vi "Set pump parameters.vi"(4 "Pump write delay (ms)":dbl=300.0, 5 "Volume (uL)":dbl, 6 "Rate (uL/h)":dbl, 7 "Units":dbl=3.0, 8 "Pump #":dbl=1.0, 9 "Pump Parameters In":T1, 10 "VISA resource name":refnum<visa-resource-name>="COM4") -> (3 "Pump Parameters Out":T1)   [LabVIEW 2014]
panel:
  out "F-format string 4":string
  out "F-format string 2":string
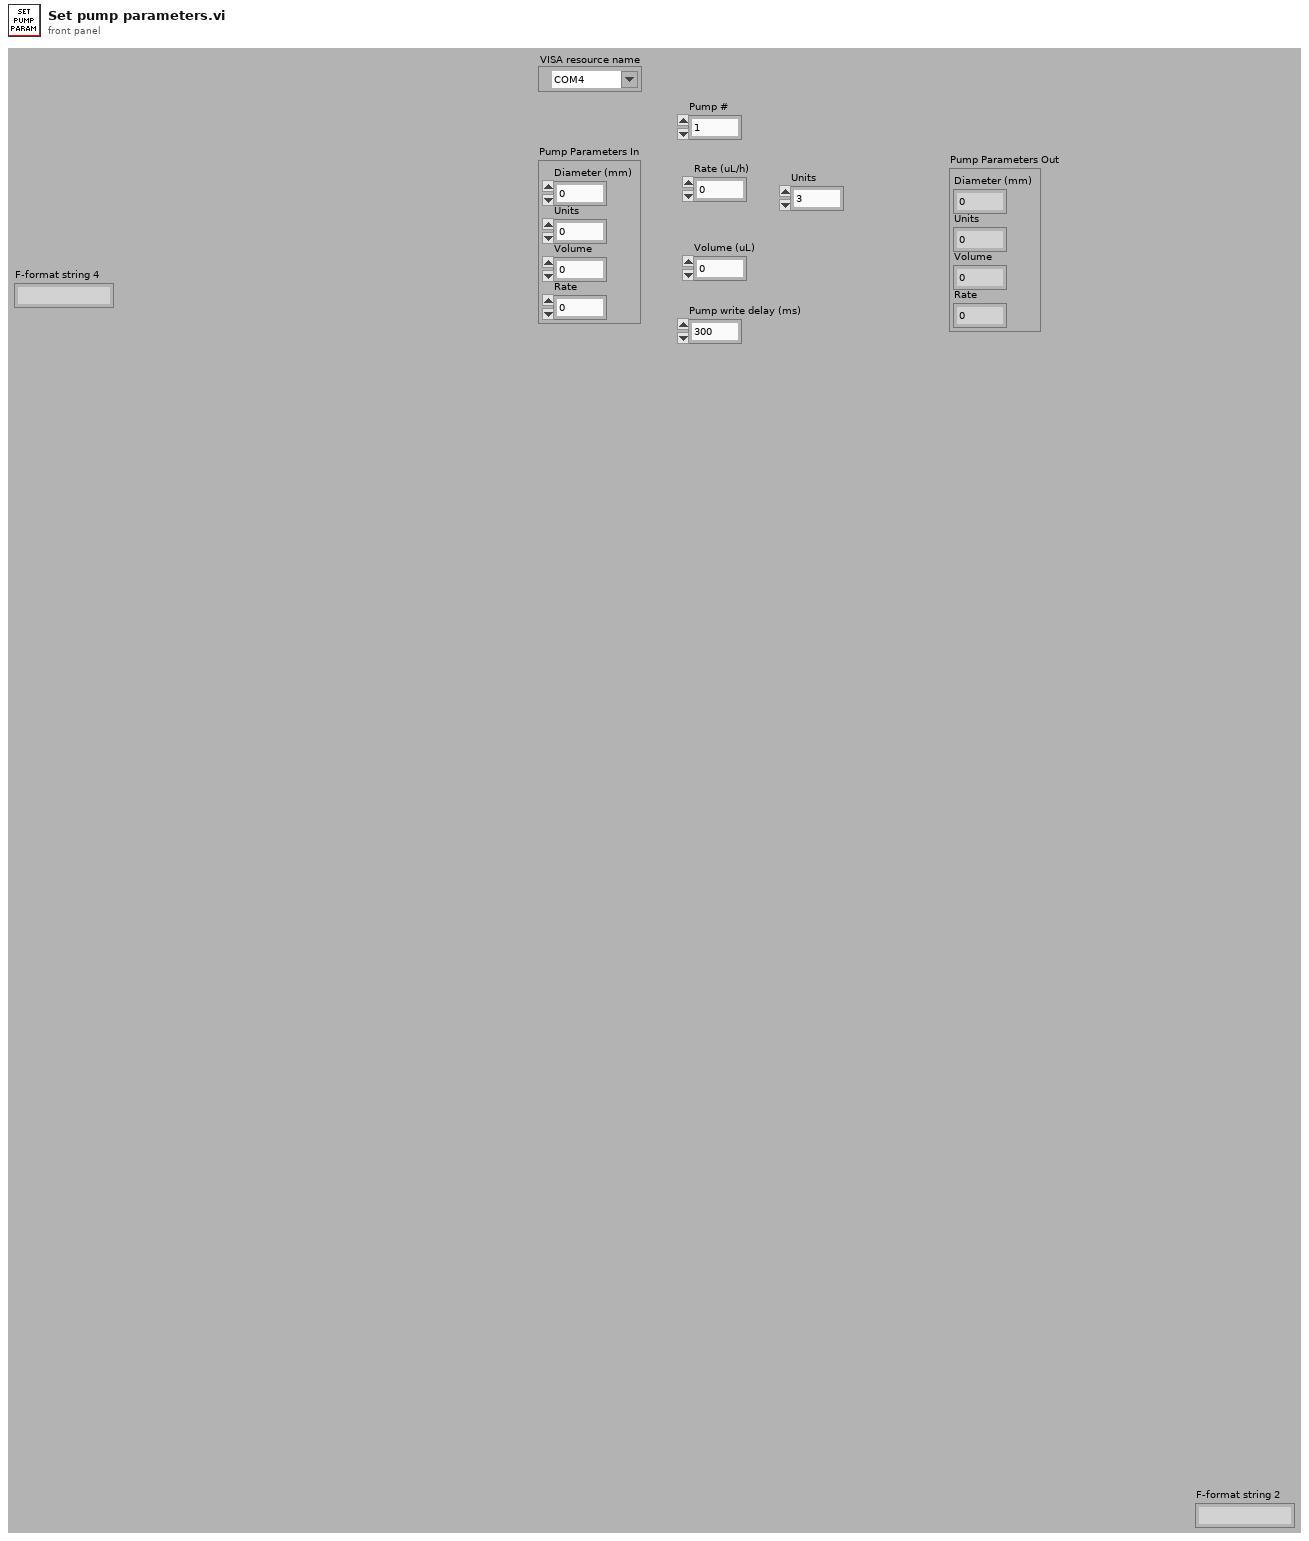
[diagram p1: front panel]
types:
  T1 = cluster{"Diameter (mm)":dbl, "Units":dbl, "Volume":dbl, "Rate":dbl}
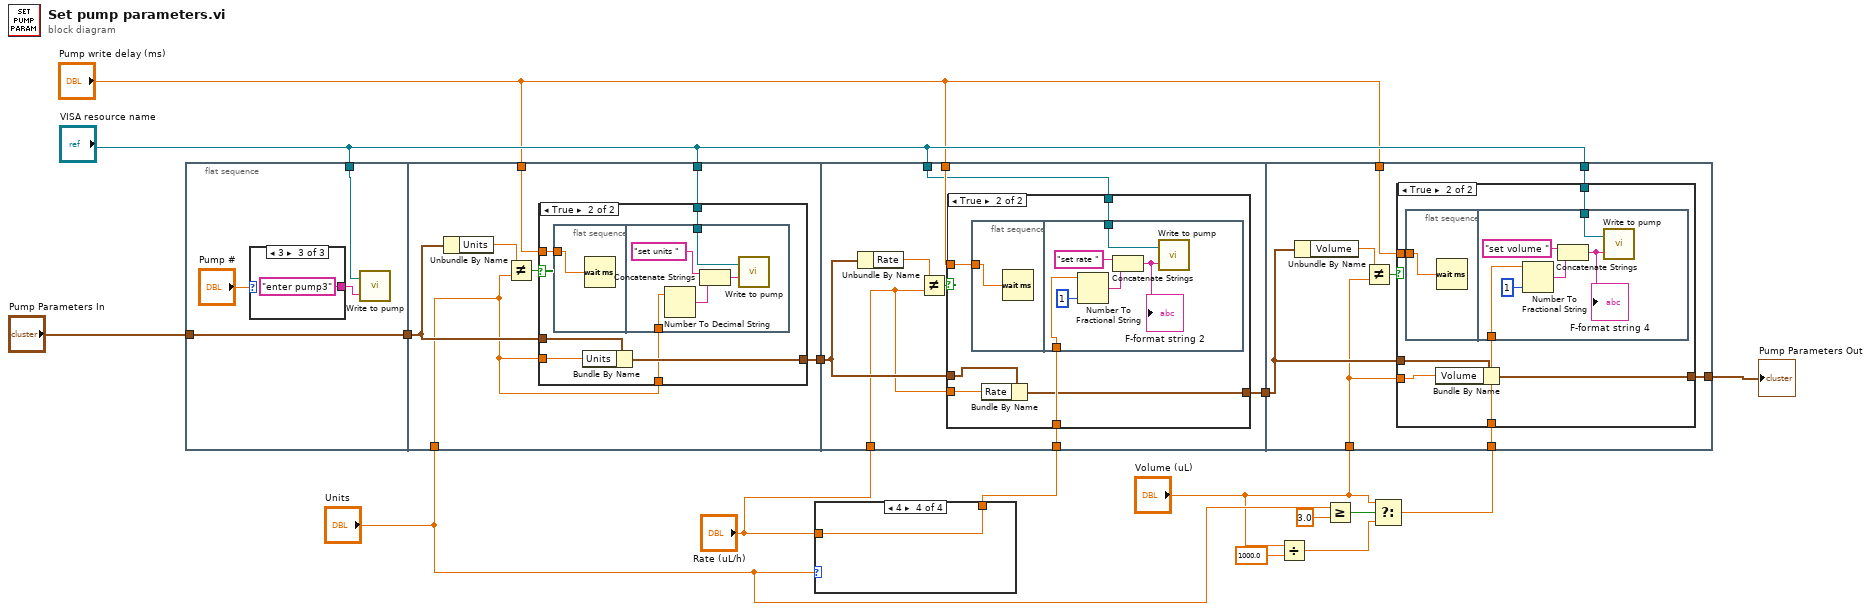
[diagram p0: block diagram]
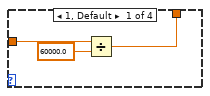
[diagram p2: hidden frame]
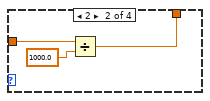
[diagram p3: hidden frame]
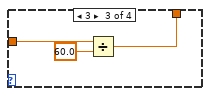
[diagram p4: hidden frame]
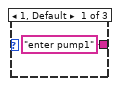
[diagram p5: hidden frame]
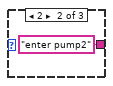
[diagram p6: hidden frame]
diagram:
  n1 = flat-sequence {
    tunnel: "VISA resource name" -> [w17]
    tunnel: [w20] -> w16
    tunnel: "Pump Parameters In" -> [w20]
    tunnel: "VISA resource name" -> [w30]
    tunnel: "Pump write delay (ms)" -> [w27]
    tunnel: w16 -> [w26]
    tunnel: [w25] -> w15
    tunnel: "Units" -> [w24]
    tunnel: "VISA resource name" -> [w45]
    tunnel: "Rate (uL/h)" -> [w47]
    tunnel: "Pump write delay (ms)" -> [w49]
    tunnel: w15 -> [w48]
    tunnel: [w46] -> w14
    tunnel: w8 -> [w44]
    tunnel: "VISA resource name" -> [w70]
    tunnel: "Volume (uL)" -> [w68]
    tunnel: "Pump write delay (ms)" -> [w71]
    tunnel: w14 -> [w69]
    tunnel: [w67] -> w10
    tunnel: w4 -> [w66]
    frame #0 {
      n2 = case shown="3" "Pump #" {
        tunnel: ["enter pump1" ("string") "enter pump2" ("string") "enter pump3" ("string")] -> w18
        frame 1, Default {
        }
        frame 2 {
        }
        frame 3 {
        }
      }
      n3 = call "Write to pump.vi"("string"=w18, "VISA resource name"=w17) -> ()  [unwired: 1 out]
    }
    frame #1 {
      n4 = Unbundle By Name(w26) -> ("Units"=w28:dbl)
      n5 = Not Equal?(x=w28, y=w24) -> (x != y?=w29:bool)
      n6 = case shown="True" w29 {
        tunnel: w30 -> [_ w37]
        tunnel: w27 -> [_ w36]
        tunnel: w26 -> [w31 w35]
        tunnel: w24 -> [_ w34]
        tunnel: [w31 w33] -> w25
        tunnel: w24 -> [_ w32]
        frame False {
        }
        frame True {
          n7 = flat-sequence {
            tunnel: w36 -> [w38]
            tunnel: w37 -> [w43]
            tunnel: w32 -> [w41]
            frame #0 {
              n8 = Wait (ms)(milliseconds to wait=w38) -> ()  [unwired: 1 out]
            }
            frame #1 {
              n9 = Number To Decimal String(number=w41) -> (decimal integer string=w42:string)  [unwired: 1 in]
              n10 = Concatenate Strings("set units " ("string"), w42) -> (w39:string)
              n11 = call "Write to pump.vi"("string"=w39, "VISA resource name"=w43) -> ()  [unwired: 1 out]
            }
          }
          n12 = Bundle By Name(cluster=w35, "Units"=w34) -> (w33:T1)
        }
      }
    }
    frame #2 {
      n13 = Unbundle By Name(w48) -> ("Rate"=w50:dbl)
      n14 = Not Equal?(x=w50, y=w47) -> (x != y?=w51:bool)
      n15 = case shown="True" w51 {
        tunnel: w49 -> [_ w58]
        tunnel: w44 -> [_ w57]
        tunnel: w48 -> [w52 w56]
        tunnel: w47 -> [_ w55]
        tunnel: [w52 w54] -> w46
        tunnel: w45 -> [_ w53]
        frame False {
        }
        frame True {
          n16 = flat-sequence {
            tunnel: w58 -> [w59]
            tunnel: w57 -> [w61]
            tunnel: w53 -> [w60]
            frame #0 {
              n17 = Wait (ms)(milliseconds to wait=w59) -> ()  [unwired: 1 out]
            }
            frame #1 {
              n18 = Number To Fractional String(number=w61, precision (6)=i16 1) -> (F-format string=w64:string)  [unwired: 2 in]
              n19 = Concatenate Strings("set rate " ("string"), w64) -> (w62:string)
              "F-format string 2" <- w62
              n20 = call "Write to pump.vi"("string"=w62, "VISA resource name"=w60) -> ()  [unwired: 1 out]
            }
          }
          n21 = Bundle By Name(cluster=w56, "Rate"=w55) -> (w54:T1)
        }
      }
    }
    frame #3 {
      n22 = Unbundle By Name(w69) -> ("Volume"=w72:dbl)
      n23 = Not Equal?(x=w72, y=w68) -> (x != y?=w73:bool)
      n24 = case shown="True" w73 {
        tunnel: w71 -> [_ w80]
        tunnel: w70 -> [_ w79]
        tunnel: w66 -> [_ w78]
        tunnel: w69 -> [w74 w77]
        tunnel: w68 -> [_ w76]
        tunnel: [w74 w75] -> w67
        frame False {
        }
        frame True {
          n25 = flat-sequence {
            tunnel: w80 -> [w81]
            tunnel: w79 -> [w83]
            tunnel: w78 -> [w82]
            frame #0 {
              n26 = Wait (ms)(milliseconds to wait=w81) -> ()  [unwired: 1 out]
            }
            frame #1 {
              n27 = Number To Fractional String(number=w82, precision (6)=i16 1) -> (F-format string=w86:string)  [unwired: 2 in]
              n28 = Concatenate Strings("set volume " ("string"), w86) -> (w84:string)
              "F-format string 4" <- w84
              n29 = call "Write to pump.vi"("string"=w84, "VISA resource name"=w83) -> ()  [unwired: 1 out]
            }
          }
          n30 = Bundle By Name(cluster=w77, "Volume"=w76) -> (w75:T1)
        }
      }
    }
  }
  n31 = case shown="4" "Units" {
    tunnel: "Rate (uL/h)" -> [w90 w92 w96 w97]
    tunnel: [w89 w93 w95 w97] -> w8
    frame 1, Default {
      n32 = Divide(x=w90, y=60000.0) -> (x/y=w89:dbl)
    }
    frame 2 {
      n33 = Divide(x=w92, y=1000.0) -> (x/y=w93:dbl)
    }
    frame 3 {
      n34 = Divide(x=w96, y=60.0) -> (x/y=w95:dbl)
    }
    frame 4 {
    }
  }
  n35 = Divide(x="Volume (uL)", y=1000.0) -> (x/y=w2:dbl)
  n36 = Greater Or Equal?(x="Units", y=3.0) -> (x >= y?=w7:bool)
  n37 = Select(t="Volume (uL)", s=w7, f=w2) -> (s? t:f=w4:dbl)
  "Pump Parameters Out" <- w10
